vi "subConfocal_visaIO.vi"(0 "VISA  IN":refnum<visa-resource-name>, 2 "Dwell Time (ms)":u32(knob)=75 scale=0.0..100.0, 5 "Communication Port":i32(ring) items=["COM", "USB"], 7 "Command (to ctlr)":string, 11 "error in":errorcluster) -> (4 "VISA OUT":refnum<visa-resource-name>, 6 "Communication Port Out":i32(ring) items=["COM", "USB"], 8 "Raw Response":string, 10 "Numeric response":string=":A 0\n", 15 "error out":errorcluster)   [LabVIEW 2015]
doc: "SubVI for sending commands to the MAC5000 and receiving responses from the MAC5000."
panel:
  out "Numeric":i32
  out "bytes to read":u32
  out "return count":u32
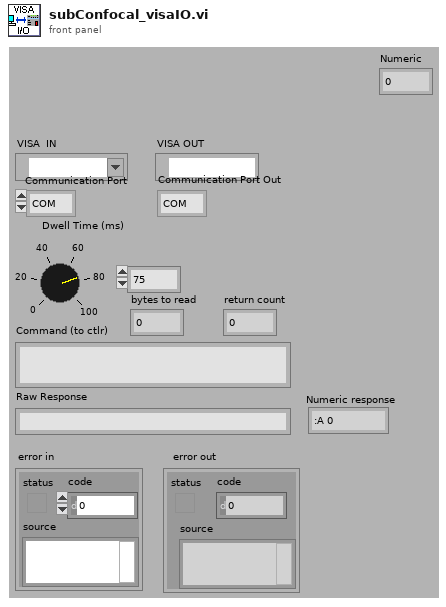
[diagram p1: front panel]
types:
  T1 = cluster{"status":bool, "code":bool, "source":bool}
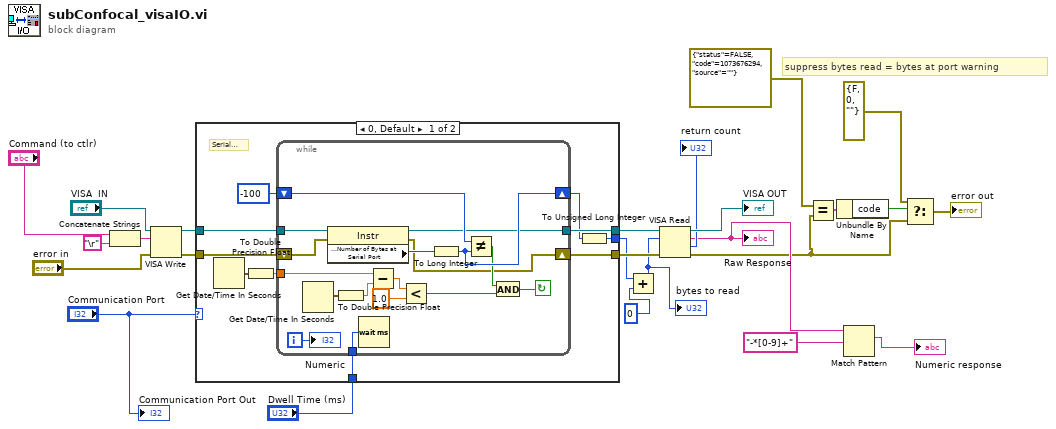
[diagram p0: block diagram]
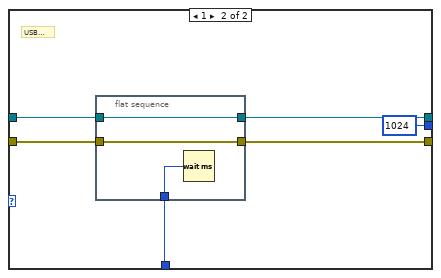
[diagram p2: hidden frame]
diagram:
  # "suppress bytes read = bytes at port warning"
  n1 = Concatenate Strings("Command (to ctlr)", "\r") -> (w14:string)
  n2 = VISA Write(VISA resource name="VISA  IN", write buffer=w14, error in (no error)="error in") -> (VISA resource name out=w24:refnum<visa-resource-name>, error out=w22:errorcluster)  [unwired: 1 out]
  n3 = case shown="0, Default" "Communication Port" {
    tunnel: w24 -> [w35 w58]
    tunnel: w22 -> [w33 w55]
    tunnel: [w30 w57] -> w21
    tunnel: [w29 w54] -> w20
    tunnel: [w28 u32 1024] -> w11
    tunnel: "Dwell Time (ms)" -> [w26 w53]
    frame 0, Default {
      # "Serial Port"
      n4 = Get Date/Time In Seconds() -> (seconds since 1Jan1904=w32:timestamp)
      n5 = To Double Precision Float(number=w32) -> (double precision float=w31:dbl)
      n6 = while {
        shift-right: [w49] -> w27
        shift-left: -100 -> [w50]
        tunnel: w35 -> [w52]
        shift-right: [w39] -> w29
        shift-left: w33 -> [w48]
        tunnel: w31 -> [w44]
        tunnel: [w46] -> w30
        tunnel: w26 -> [w37]
        i -> [w36]
        stop <- w38 continue-if-true
        n7 = Get Date/Time In Seconds() -> (seconds since 1Jan1904=w47:timestamp)
        n8 = property class="Instr"(reference=w52, error in=w48) -> (reference out=w46:refnum<visa-resource-name>, error out=w39:errorcluster, "Serial Settings:Number of Bytes at Serial Port"=w51:u32)
        n9 = To Double Precision Float(number=w47) -> (double precision float=w45:dbl)
        n10 = Wait (ms)(milliseconds to wait=w37) -> ()  [unwired: 1 out]
        n11 = Subtract(x=w44, y=w45) -> (x-y=w43:dbl)
        n12 = Less?(x=w43, y=1.0) -> (x < y?=w41:bool)
        n13 = To Long Integer(number=w51) -> (32bit integer=w49:i32)
        n14 = Not Equal?(x=w50, y=w49) -> (x != y?=w40:bool)
        n15 = And(x=w40, y=w41) -> (x .and. y?=w38:bool)
        "Numeric" <- w36
      }
      n16 = To Unsigned Long Integer(number=w27) -> (unsigned 32bit integer=w28:u32)
    }
    frame 1 {
      # "USB Port"
      n17 = flat-sequence {
        tunnel: w58 -> [w61]
        tunnel: [w61] -> w57
        tunnel: w55 -> [w60]
        tunnel: [w60] -> w54
        tunnel: w53 -> [w59]
        frame #0 {
          n18 = Wait (ms)(milliseconds to wait=w59) -> ()  [unwired: 1 out]
        }
      }
    }
  }
  n19 = Add(x=w11, y=0) -> (x+y=w10:u32)
  "bytes to read" <- w10
  n20 = VISA Read(VISA resource name=w21, byte count=w10, error in (no error)=w20) -> (VISA resource name out=→"VISA OUT":refnum<visa-resource-name>, read buffer=w7:string, return count=→"return count":u32, error out=w2:errorcluster)
  "Raw Response" <- w7
  n21 = Equal?(x=errorcluster {"status"=FALSE, "code"=1073676294, "source"=""}, y=w2) -> (x = y?=w5:T1)
  n22 = Unbundle By Name(w5) -> ("code"=w4:bool)
  n23 = Match Pattern(string=w7, regular expression="-*[0-9]+") -> (match substring=→"Numeric response":string)  [unwired: 1 in, 3 out]
  n24 = Select(t=errorcluster {"status"=FALSE, "code"=0, "source"=""} ("x"), s=w4, f=w2) -> (s? t:f=→"error out":errorcluster)
  "Communication Port Out" <- "Communication Port"
